vi "Configure Tester Dialog.vi"(7 "Console Log in":refnum<class "Console Log.lvclass">, 8 "error in":errorcluster, 11 "Potting Procedure In":refnum<class "Potting Procedure.lvclass">) -> (0 "error out":errorcluster, 2 "Canceled":bool, 3 "Potting Procedure Out":refnum<class "Potting Procedure.lvclass">, 5 "Console Log out":refnum<class "Console Log.lvclass">)   [LabVIEW 2017]
uses:
  UI typedefs/Chuck Slot Control.ctl
  UI typedefs/Chuck Control.ctl
  Procedure Classes/Potting Procedure/Type Definitions/Configure Tester.ctl
  Procedure Classes/Potting Procedure/Potting Procedure.lvclass
  Shared Components/WorkTable Class/WorkTable Class.lvclass
  Application Utilities/Console Log/Console Log.lvclass
panel:
  in  "Module Chuck 5":T1
  in  "Module Chuck 4":T1
  in  "Module Chuck 3":T1
  in  "Module Chuck 2":T1
  in  "Module Chuck 1":T1
  in  "OK Button":bool
  in  "Cancel Button":bool
  # "INSTRUCTIONS\n\nClick inside the boxes to indicate whether\na slot is populated.\n\nFor each populated chuck enter the serial\nnumber in the provided text field."
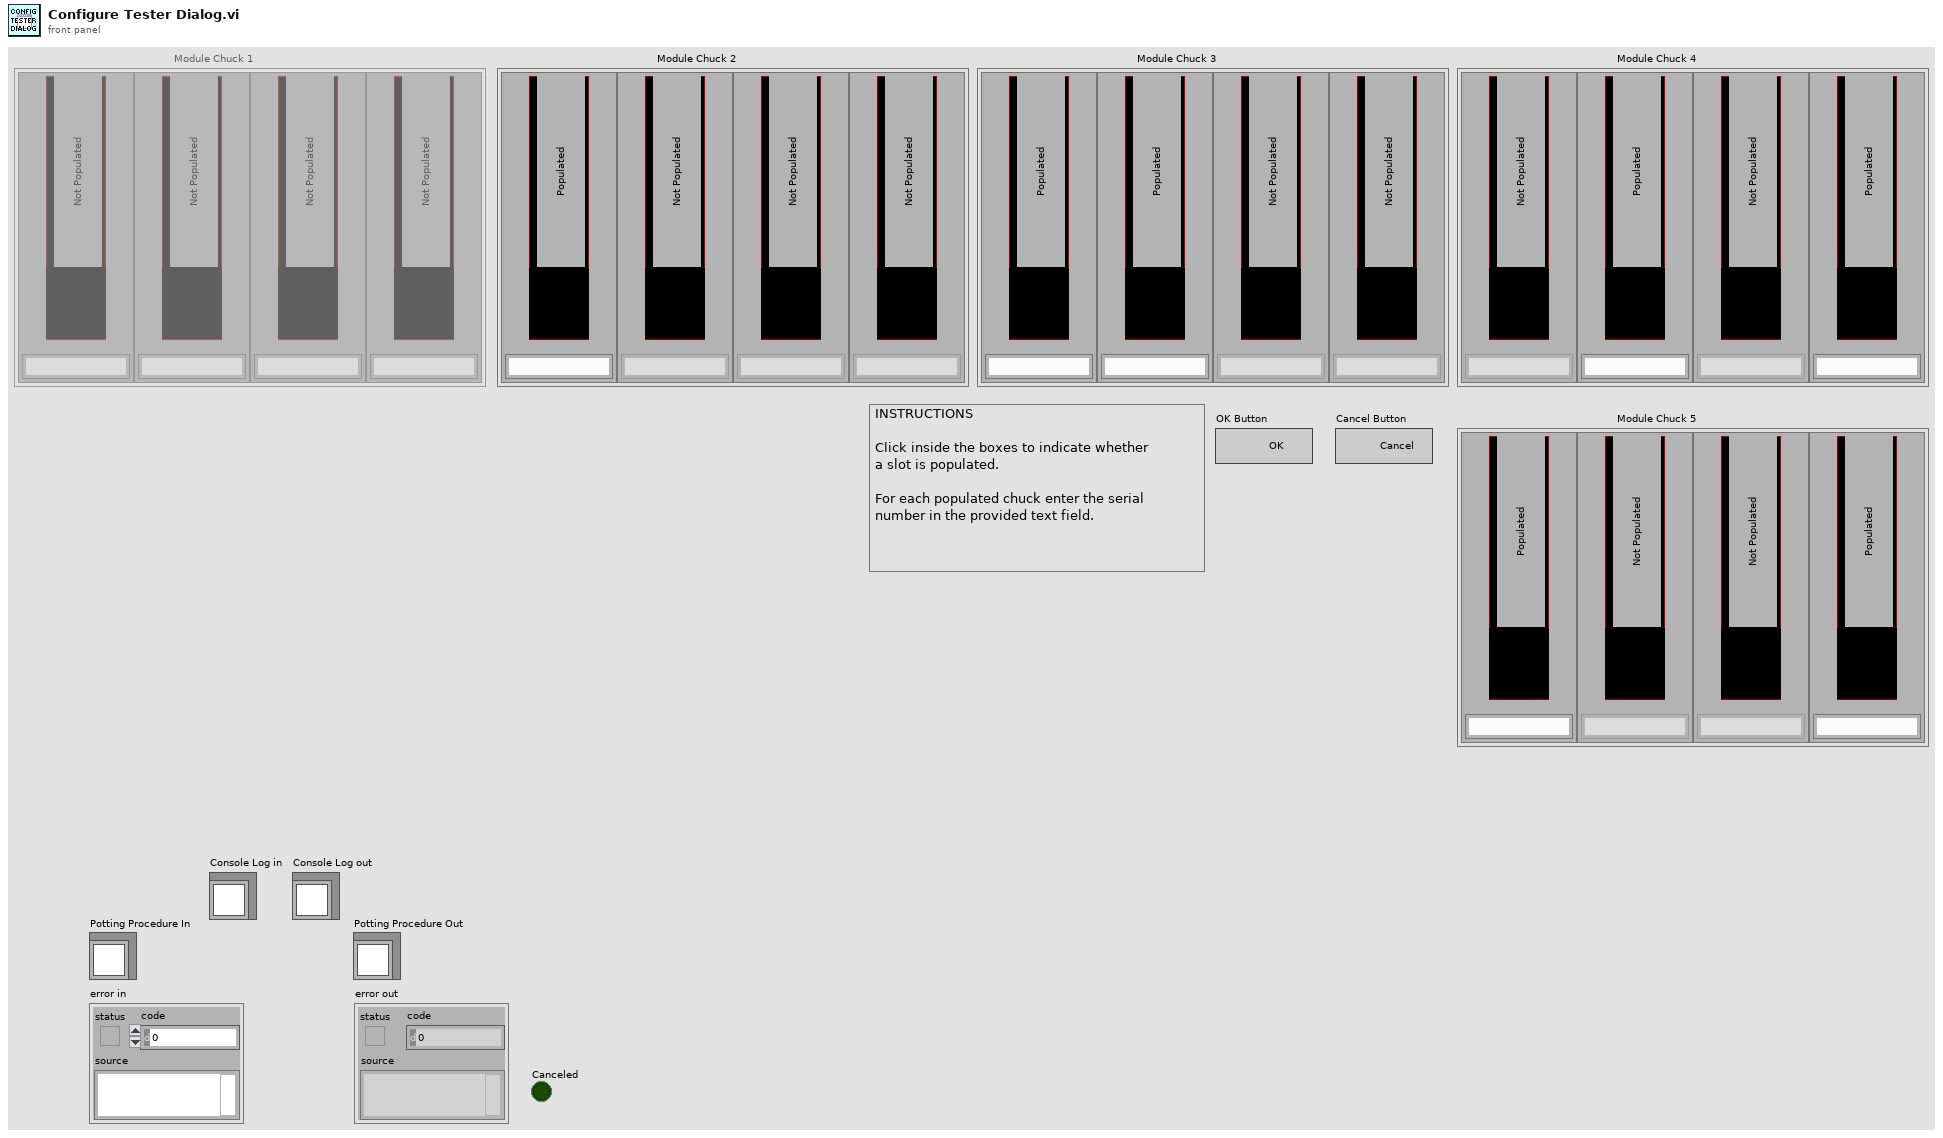
[diagram p1: front panel]
types:
  T1 = typedef "Chuck Control.ctl" = cluster{"Slot 1":T2, "Slot 2":T2, "Slot 3":T2, "Slot 4":T2}
  T2 = typedef "Chuck Slot Control.ctl" = cluster{"Slot Populated":bool, "S/N":string}
  T3 = enum8{"Enabled", "Disabled", "Disabled and Grayed Out"}
  T4 = enum16{"Empty", "Bare HDI", "Unglued", "Stamped", "PartOnTop", "Weighted", "Unpotted", "Potted"}
  T5 = typedef "Worktable_Module Slot.ctl" = cluster{"Slot State":enum16{"Empty", "Bare HDI", "Unglued", "Stamped", "PartOnTop", "Weighted", "Unpotted", "Potted"}, "BBM Type":enum16{"None", "BBM", "GlassSlide"}, "HDI Type":enum16{"None", "HDI", "Polyimide"}, "Vacuum Channel":u8, "Location/Orientation BBM":T6, "Location/Orientation HDI":T6, "S/N":string}
  T6 = typedef "Position_Orientation.ctl" = cluster{"Center":refnum<class "Vec3d Class.lvclass">, "Orientation":refnum<class "Orient3d Class.lvclass">}
  T7 = typedef "Configure Tester.ctl" = cluster{"Has Been Run?":bool}
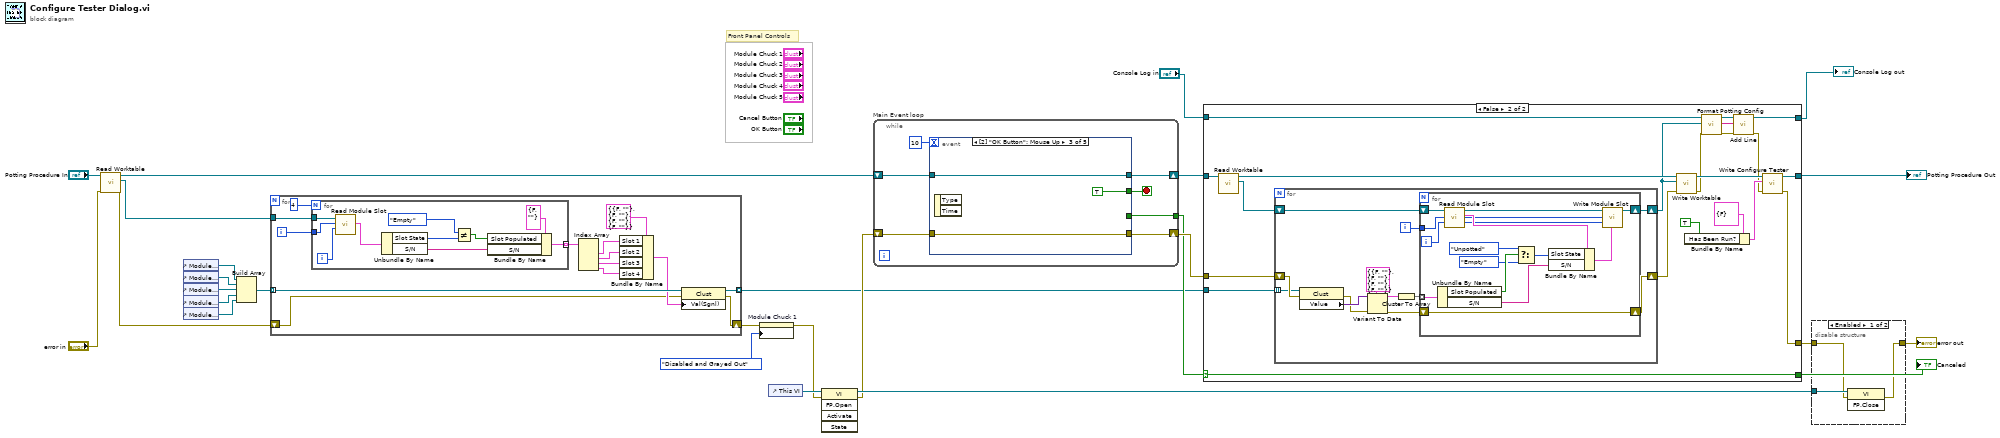
[diagram p0: block diagram]
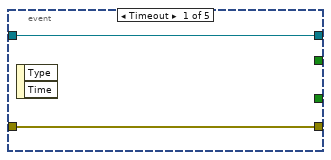
[diagram p4: hidden frame]
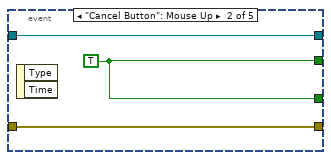
[diagram p5: hidden frame]
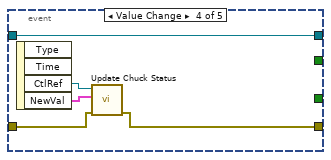
[diagram p6: hidden frame]
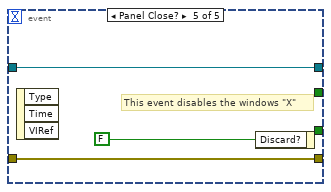
[diagram p7: hidden frame]
diagram:
  # "Front Panel Controls"
  n1 = call-dynamic "Read Worktable.vi"("error in"="error in", "Potting Procedure in"="Potting Procedure In") -> ("error out"=w6:errorcluster, "WorkTable out"=w7:refnum<class "WorkTable Class.lvclass">, "Potting Procedure out"=w19:refnum<class "Potting Procedure.lvclass">)  [unwired: 7 in]
  n2 = control-ref of="Module Chuck 1"() -> (w12:refnum<vi>)
  n3 = control-ref of="Module Chuck 2"() -> (w11:refnum<vi>)
  n4 = control-ref of="Module Chuck 3"() -> (w10:refnum<vi>)
  n5 = control-ref of="Module Chuck 4"() -> (w9:refnum<vi>)
  n6 = control-ref of="Module Chuck 5"() -> (w8:refnum<vi>)
  n7 = Build Array(w12, w11, w10, w9, w8) -> (w4:refnum<vi>[])
  n8 = for {
    tunnel: w4 -> [w34] mode=indexing
    shift-right: [w32] -> w5
    shift-left: w6 -> [w31]
    tunnel: w7 -> [w29]
    tunnel: [w30] -> w3 mode=indexing
    i -> [w28]
    n9 = for {
      N: 4 -> [_]
      tunnel: [w49] -> w39 mode=indexing
      tunnel: w29 -> [w46]
      tunnel: w28 -> [w44]
      i -> [w45]
      n10 = call-dynamic "Read Module Slot.vi"("slot"=w45, "chuck"=w44, "WorkTable in"=w46) -> ("Module Slot"=w43:T5)  [unwired: 6 in, 2 out]
      n11 = Unbundle By Name(w43) -> ("Slot State"=w48:T4, "S/N"=w47:string)
      n12 = Not Equal?(x=T4."Empty" ("Slot State"), y=w48) -> (x != y?=w50:bool)
      n13 = Bundle By Name(cluster=T2 {"Slot Populated"=FALSE, "S/N"=""} ("Slot 1"), "Slot Populated"=w50, "S/N"=w47) -> (w49:T2)
    }
    n14 = Index Array(array=w39) -> (element #1=w38:T2, element #2=w37:T2, element #3=w36:T2, element #4=w35:T2)  [unwired: 4 in]
    n15 = Bundle By Name(cluster=T1 {"Slot 1"={"Slot Populated"=FALSE, "S/N"=""}, "Slot 2"={"Slot Populated"=FALSE, "S/N"=""}, "Slot 3"={"Slot Populated"=FALSE, "S/N"=""}, "Slot 4"={"Slot Populated"=FALSE, "S/N"=""}} ("BBM Chuck 1"), "Slot 1"=w38, "Slot 2"=w37, "Slot 3"=w36, "Slot 4"=w35) -> (w33:T1)
    n16 = property class="Clust"(reference=w34, error in=w31, "Val(Sgnl)"=w33) -> (reference out=w30:refnum<vi>, error out=w32:errorcluster)
  }
  n17 = property on="Module Chuck 1" class="Clust"(error in=w5, "DisabledEnum"=T3."Disabled and Grayed Out" ("Disabled")) -> (error out=w14:errorcluster)  [unwired: 1 in, 1 out]
  n18 = control-ref of="This VI"() -> (w27:refnum<vi>)
  n19 = invoke class="VI" method="FP.Open"(reference=w27, error in=w14) -> (reference out=w26:refnum<vi>, error out=w24:errorcluster)  [unwired: 3 in, 3 out]
  n20 = while "Main Event loop" {
    tunnel: [w54] -> w16
    shift-right: [w52] -> w22
    shift-left: w19 -> [w53]
    shift-right: [w56] -> w18
    shift-left: w24 -> [w55]
    stop <- w57 stop-if-true
    n21 = event shown="[2] \"OK Button\": Mouse Up" {
      selector: _ -> [_ _ _ _ _]
      dyn-events: _ -> [_ _ _ _ _]
      timeout: 10 -> [_ _ _ _ _]
      tunnel: [_ w62 TRUE _ _] -> w57
      tunnel: [w60 w63 w66 w67 w73] -> w56
      tunnel: w55 -> [w60 w63 w66 w70 w73]
      tunnel: [_ w62 _ _ _] -> w54
      tunnel: w53 -> [w59 w61 w64 w68 w72]
      tunnel: [w59 w61 w64 w68 w72] -> w52
      event Timeout {
        n22 = event-data() -> ()  [unwired: 1 in, 2 out]
      }
      event "Cancel Button": Mouse Up {
        w62 = TRUE
        n23 = event-data() -> ()  [unwired: 1 in, 2 out]
      }
      event "OK Button": Mouse Up {
        n24 = event-data() -> ()  [unwired: 1 in, 2 out]
      }
      event Value Change {
        n25 = event-data() -> ("CtlRef"=w71:refnum<vi>, "NewVal"=w69:T1)  [unwired: 1 in, 2 out]
        n26 = call "Update Chuck Status.vi"("error in"=w70, "Chuck Value"=w69, "Chuck Reference In"=w71) -> ("error out"=w67:errorcluster)  [unwired: 8 in]
      }
      event Panel Close? {
        # "This event disables the windows \"X\""
        n27 = event-data() -> ()  [unwired: 1 in, 3 out]
        n28 = event-data("Discard?"=FALSE) -> ()  [unwired: 1 in, 1 out]
      }
    }
  }
  n29 = case shown="False" w16 {
    selector: w16 -> [w76 w94]
    tunnel: w22 -> [w78 w93]
    tunnel: [w78 w99] -> w21
    tunnel: w18 -> [w77 w88]
    tunnel: [w77 w96] -> w17
    tunnel: [w76 w94] -> w13
    tunnel: w3 -> [_ w87]
    tunnel: "Console Log in" -> [w75 w85]
    tunnel: [w75 w81] -> w1
    frame True {
    }
    frame False {
      n30 = call-dynamic "Read Worktable.vi"("Potting Procedure in"=w93) -> ("WorkTable out"=w92:refnum<class "WorkTable Class.lvclass">, "Potting Procedure out"=w91:refnum<class "Potting Procedure.lvclass">)  [unwired: 8 in, 1 out]
      n31 = for {
        shift-right: [w106] -> w86
        shift-left: w92 -> [w108]
        shift-right: [w104] -> w89
        shift-left: w88 -> [w103]
        tunnel: w87 -> [w100] mode=indexing
        i -> [w107]
        n32 = property class="Clust"(reference=w100, error in=w103) -> (error out=w101:errorcluster, "Value"=w102:variant)  [unwired: 1 out]
        n33 = Variant To Data(error in=w101, type=T1 {"Slot 1"={"Slot Populated"=FALSE, "S/N"=""}, "Slot 2"={"Slot Populated"=FALSE, "S/N"=""}, "Slot 3"={"Slot Populated"=FALSE, "S/N"=""}, "Slot 4"={"Slot Populated"=FALSE, "S/N"=""}} ("BBM Chuck 1"), Variant=w102) -> (data=w110:T1, error out=w105:errorcluster)
        n34 = Cluster To Array(cluster=w110) -> (array=w109:T2[])
        n35 = for {
          tunnel: w109 -> [w125] mode=indexing
          tunnel: w107 -> [w120]
          shift-right: [w118] -> w106
          shift-left: w108 -> [w116]
          shift-right: [w117] -> w104
          shift-left: w105 -> [w117]
          i -> [w121]
          n36 = Unbundle By Name(w125) -> ("Slot Populated"=w123:bool, "S/N"=w124:string)
          n37 = call-dynamic "Read Module Slot.vi"("slot"=w121, "chuck"=w120, "WorkTable in"=w116) -> ("Module Slot"=w122:T5, "WorkTable out"=w115:refnum<class "WorkTable Class.lvclass">)  [unwired: 6 in, 1 out]
          n38 = Select(t=T4."Unpotted" ("Slot State"), s=w123, f=T4."Empty" ("Slot State")) -> (s? t:f=w112:T4)
          n39 = Bundle By Name(cluster=w122, "Slot State"=w112, "S/N"=w124) -> (w119:T5)
          n40 = call-dynamic "Write Module Slot.vi"("Module Slot"=w119, "slot"=w121, "chuck"=w120, "WorkTable in"=w115) -> ("WorkTable out"=w118:refnum<class "WorkTable Class.lvclass">)  [unwired: 6 in, 1 out]
        }
      }
      n41 = call-dynamic "Write Worktable.vi"("error in"=w89, "WorkTable in"=w86, "Potting Procedure in"=w91) -> ("error out"=w80:errorcluster, "Potting Procedure out"=w90:refnum<class "Potting Procedure.lvclass">)  [unwired: 7 in]
      n42 = Bundle By Name(cluster=T7 {"Has Been Run?"=FALSE} ("Configure Tester"), "Has Been Run?"=TRUE) -> (w97:T7)
      n43 = call "Format Potting Config.vi"("error in"=w80, "Worktable"=w86, "Console Log in"=w85) -> ("error out"=w84:errorcluster, "Formatted Worktable Config"=w83:string, "Console Log out"=w82:refnum<class "Console Log.lvclass">)  [unwired: 6 in]
      n44 = call "Add Line.vi"("error in"=w84, "String"=w83, "Console Log in"=w82) -> ("error out"=w79:errorcluster, "Console Log out"=w81:refnum<class "Console Log.lvclass">)  [unwired: 7 in]
      n45 = call-dynamic "Write Configure Tester.vi"("error in (no error)"=w79, "Configure Tester"=w97, "Potting Procedure in"=w90) -> ("error out"=w96:errorcluster, "Potting Procedure out"=w99:refnum<class "Potting Procedure.lvclass">)  [unwired: 7 in]
    }
  }
  "Canceled" <- w13
  "Potting Procedure Out" <- w21
  "Console Log out" <- w1
  n46 = disable-structure shown="Enabled" {
    disable-tunnel: w26 -> [w128 _]
    disable-tunnel: [w127 w129] -> w25
    disable-tunnel: w17 -> [w126 w129]
    frame Enabled {
      n47 = invoke class="VI" method="FP.Close"(reference=w128, error in=w126) -> (error out=w127:errorcluster)  [unwired: 1 in, 2 out]
    }
    frame Disabled {
    }
  }
  "error out" <- w25
